vi "SynchronizeAlgorithm.vi"(0 "xpixels":dbl, 5 "fill factor":dbl, 7 "ms/line":dbl, 9 "maximum timebase frequency":dbl, 11 "Detector maximum sampling rate":dbl, 12 "tolerance":dbl=0.1) -> (4 "Output Cluster":T1 {"Detector Timebase divisor" format="%#_4f"; "Detector Read rate" format="%#_4f"; "Actual samples to Read per Line" format="%#_4f"; "Trash Samples" format="%#_4f"; "Samples to Average" format="%#_4f"; "total pixels per line" format="%#_4f"; "Galvo Timebase divisor" format="%#_4f"; "Galvo Write rate" format="%#_4f"; "Lines/sec" format="%#_4f"; "Flyback Pixels" format="%#_4f"; "Fill Factor" format="%#_4f"; "Pixel Dwell Time (us)" format="%#_4f"; "Pixels/sec" format="%#_4f"}, 6 "iterations":i32)   [LabVIEW 2012]
uses:
  typedefs/SyncAlgo.ctl
panel:
  in  "Definition Cluster":T1 {"Detector Timebase divisor" format="%#_4f"; "Detector Read rate" format="%#_4f"; "Actual samples to Read per Line" format="%#_4f"; "Trash Samples" format="%#_4f"; "Samples to Average" format="%#_4f"; "total pixels per line" format="%#_4f"; "Galvo Timebase divisor" format="%#_4f"; "Galvo Write rate" format="%#_4f"; "Lines/sec" format="%#_4f"; "Flyback Pixels" format="%#_4f"; "Fill Factor" format="%#_4f"; "Pixel Dwell Time (us)" format="%#_4f"; "Pixels/sec" format="%#_4f"}
  out "total pixels per line":dbl format="%#_4f"
  out "Pixel Dwell Time (us)":dbl format="%#_4f"
  # "Synchronizing algorithm"
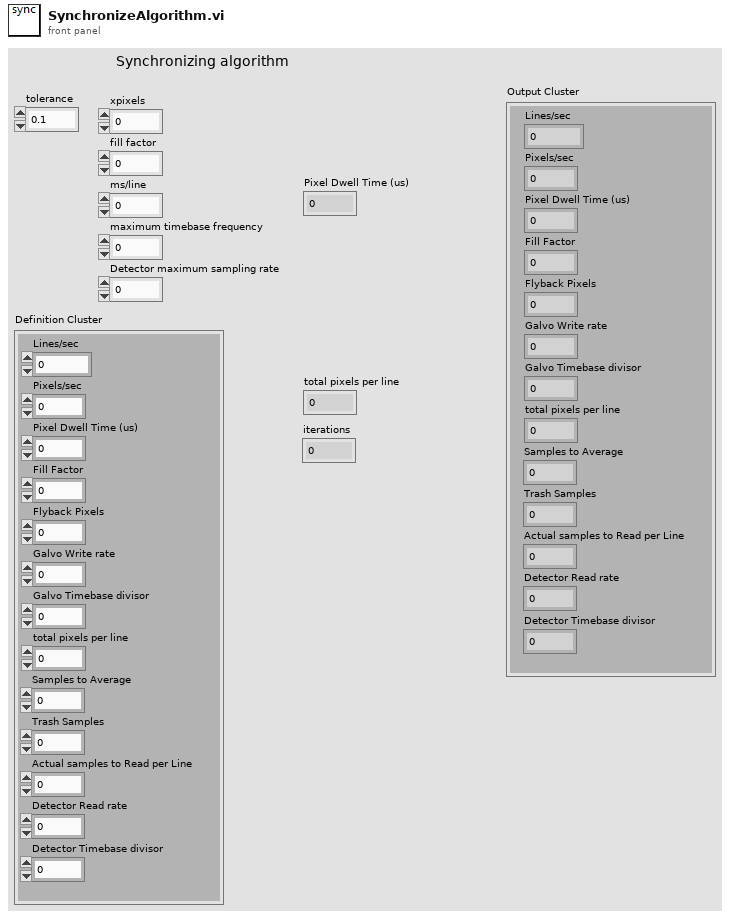
[diagram p1: front panel]
types:
  T1 = typedef "SyncAlgo.ctl" = cluster{"Pixels/sec":dbl, "Pixel Dwell Time (us)":dbl, "Fill Factor":dbl, "Flyback Pixels":dbl, "Lines/sec":dbl, "Galvo Write rate":dbl, "Galvo Timebase divisor":i32, "total pixels per line":dbl, "Samples to Average":dbl, "Trash Samples":dbl, "Actual samples to Read per Line":dbl, "Detector Read rate":dbl, "Detector Timebase divisor":i32}
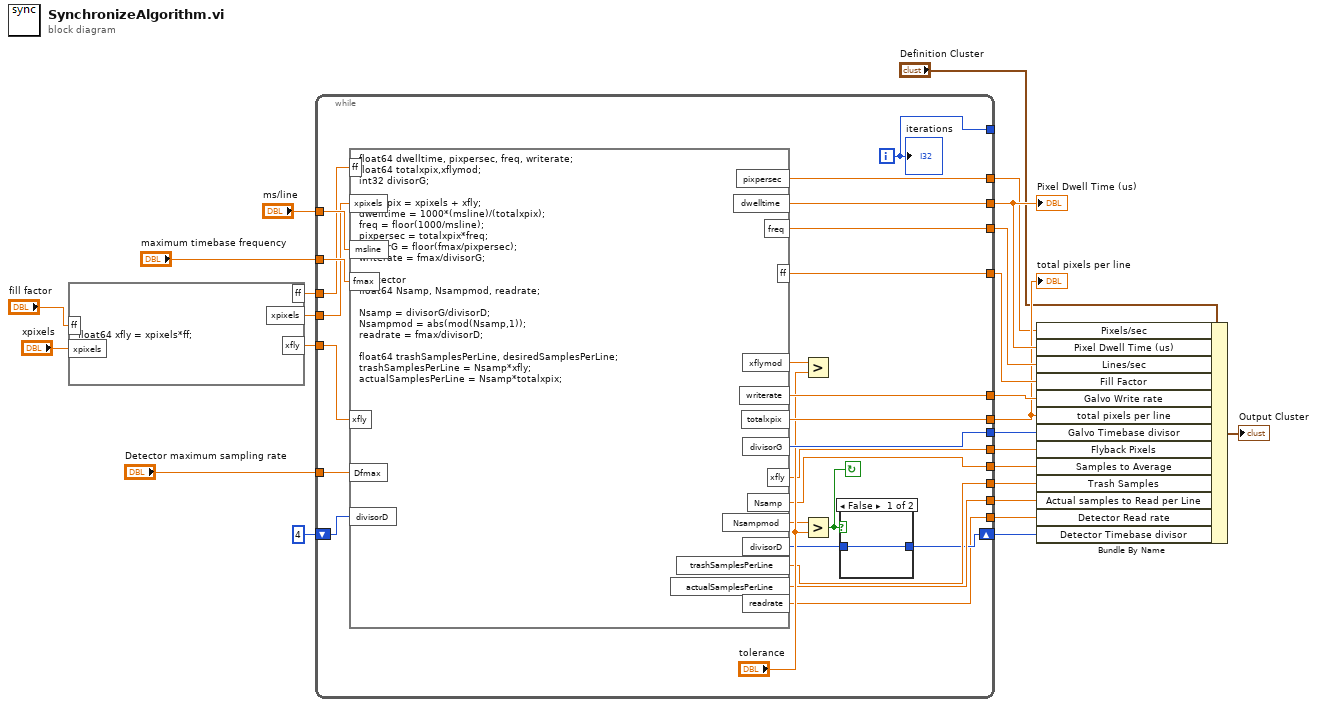
[diagram p0: block diagram]
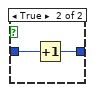
[diagram p2: hidden frame]
diagram:
  n1 = formula code="float64 xfly = xpixels*ff;"("ff"="fill factor", "xpixels"="xpixels") -> ("xfly"=w18:dbl, "xpixels"=w19:dbl, "ff"=w20:dbl)
  n2 = while {
    tunnel: "maximum timebase frequency" -> [w50]
    tunnel: "ms/line" -> [w49]
    tunnel: [w48] -> w8
    tunnel: [w47] -> w17
    tunnel: [w46] -> w16
    tunnel: [w44] -> w14
    tunnel: [w43] -> w12
    tunnel: [w42] -> w13
    tunnel: w20 -> [w41]
    tunnel: w19 -> [w40]
    tunnel: [w38] -> w15
    tunnel: [w37] -> _
    tunnel: "Detector maximum sampling rate" -> [w36]
    tunnel: [w33] -> w6
    tunnel: [w32] -> w5
    tunnel: w18 -> [w39]
    tunnel: [w31] -> w11
    tunnel: [w27] -> w4
    shift-right: [w28] -> w1
    shift-left: 4 ("divisorD") -> [w26]
    tunnel: [w25] -> w2
    i -> [w37]
    stop <- w30 continue-if-true
    n3 = formula code="float64 dwelltime, pixpersec, freq, writerate;\nfloat64 totalxpix,xflymod;\nint32 divisorG;\n\ntotalxpix = xpixels + xfly;\ndwelltime = 1000*(msline)/(totalxpix);\nfreq = floor(1000/msline);\npixpersec = totalxpix*freq;\ndivisorG = floor(fmax/pixpersec);\nwriterate = fmax/divisorG;\n\n//detector\nfloat64 Nsamp, Nsampmod, readrate;\n\nNsamp = divisorG/divisorD;\nNsampmod = abs(mod(Nsamp,1));\nreadrate = fmax/divisorD;\n\nfloat64 trashSamplesPerLine, desiredSamplesPerLine;\ntrashSamplesPerLine = Nsamp*xfly;\nactualSamplesPerLine = Nsamp*totalxpix;"("xpixels"=w40, "ff"=w41, "msline"=w49, "fmax"=w50, "xfly"=w39, "Dfmax"=w36, "divisorD"=w26) -> ("xfly"=w31:dbl, "pixpersec"=w48:dbl, "dwelltime"=w47:dbl, "ff"=w38:dbl, "freq"=w46:dbl, "xflymod"=w45:dbl, "writerate"=w44:dbl, "divisorG"=w43:i32, "totalxpix"=w42:dbl, "Nsamp"=w27:dbl, "Nsampmod"=w34:dbl, "trashSamplesPerLine"=w33:dbl, "actualSamplesPerLine"=w32:dbl, "divisorD"=w29:i32, "readrate"=w25:dbl)
    n4 = Greater?(x=w45, y="tolerance") -> ()  [unwired: 1 out]
    n5 = Greater?(x=w34, y="tolerance") -> (0:w30:bool)
    n6 = case shown="False" w30 {
      tunnel: w29 -> [w51 w53]
      tunnel: [w51 w52] -> w28
      frame False {
      }
      frame True {
        n7 = Increment(x=w53) -> (x+1=w52:i32)
      }
    }
    "iterations" <- w37
  }
  "Pixel Dwell Time (us)" <- w17
  "total pixels per line" <- w13
  n8 = Bundle By Name(cluster="Definition Cluster", "Pixels/sec"=w8, "Pixel Dwell Time (us)"=w17, "Lines/sec"=w16, "Fill Factor"=w15, "Galvo Write rate"=w14, "total pixels per line"=w13, "Galvo Timebase divisor"=w12, "Flyback Pixels"=w11, "Samples to Average"=w4, "Trash Samples"=w6, "Actual samples to Read per Line"=w5, "Detector Read rate"=w2, "Detector Timebase divisor"=w1) -> (→"Output Cluster":T1)
